vi "emi_Is Error or Warning.vi"(14 "error in (no error)":errorcluster) -> (3 "error out":errorcluster, 8 "Is Warning or Error":bool)   [LabVIEW 2010]
doc: "Extracts teh error status from error cluster,\n \n\nSaves Diagram space at teh expence of execution speed."
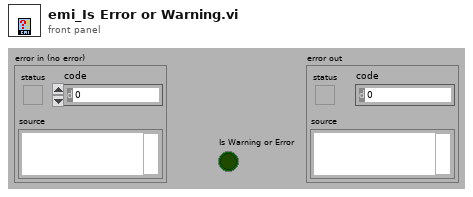
[diagram p1: front panel]
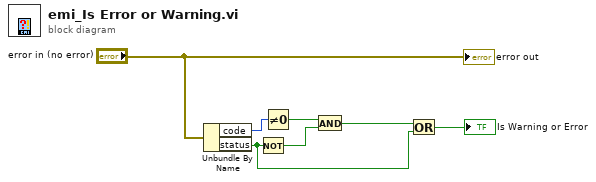
[diagram p0: block diagram]
diagram:
  n1 = Unbundle By Name("error in (no error)") -> ("code"=w7:i32, "status"=w1:bool)
  n2 = Not(x=w1) -> (.not. x?=w6:bool)
  n3 = Not Equal To 0?(x=w7) -> (x != 0?=w5:bool)
  n4 = And(x=w5, y=w6) -> (x .and. y?=w3:bool)
  n5 = Or(x=w3, y=w1) -> (x .or. y?=→"Is Warning or Error":bool)
  "error out" <- "error in (no error)"
